vi "XY with TipTilt Z.vi"() -> ()   [LabVIEW 2012]
uses:
  Madlib.dll
panel:
  in  "X axis":dbl caption="X axis (um)" format="%.3f"
  in  "Y axis (um)":dbl format="%.3f"
  in  "?":bool
  out "Read Theta A 2":dbl format="%.3f"
  out "Read Theta B 2":dbl format="%.3f"
  out "Min. Z-Axis (um)":dbl format="%.4f"
  out "Max. Z-Axis (um)":dbl format="%.4f"
  out "Theta Y (mrad)":dbl format="%.4f"
  out "Theta X (mrad)":dbl format="%.4f"
  in  "Theta Y (mrad)":dbl format="%.4f"
  out "Center (um)":dbl format="%.4f"
  in  "Z axis (um)":dbl=50.0 format="%.4f"
  in  "Theta X (mrad)":dbl format="%.4f"
  out "Min. Theta Y (mrad)":dbl format="%.4f"
  out "Max. Theta Y (mrad)":dbl format="%.4f"
  out "Min. Theta X (mrad)":dbl format="%.4f"
  out "Max. Theta X (mrad)":dbl format="%.4f"
  out "Read Theta C":dbl caption="C (um)" format="%.3f"
  out "Read Theta B":dbl caption="B (um)" format="%.3f"
  out "Read Theta A":dbl caption="A (um)" format="%.3f"
  in  "?":bool
  # "Note: You will need to obtain a handle to each controller\nusing GetHandleByType.vi to distinguish between the \ncontrollers. The initial type values passed to this VI  may\n have to be changed to work with your controllers."
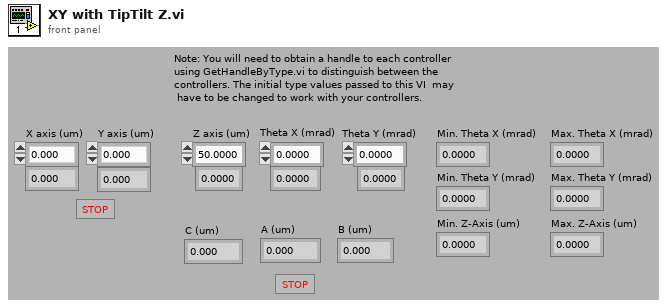
[diagram p1: front panel]
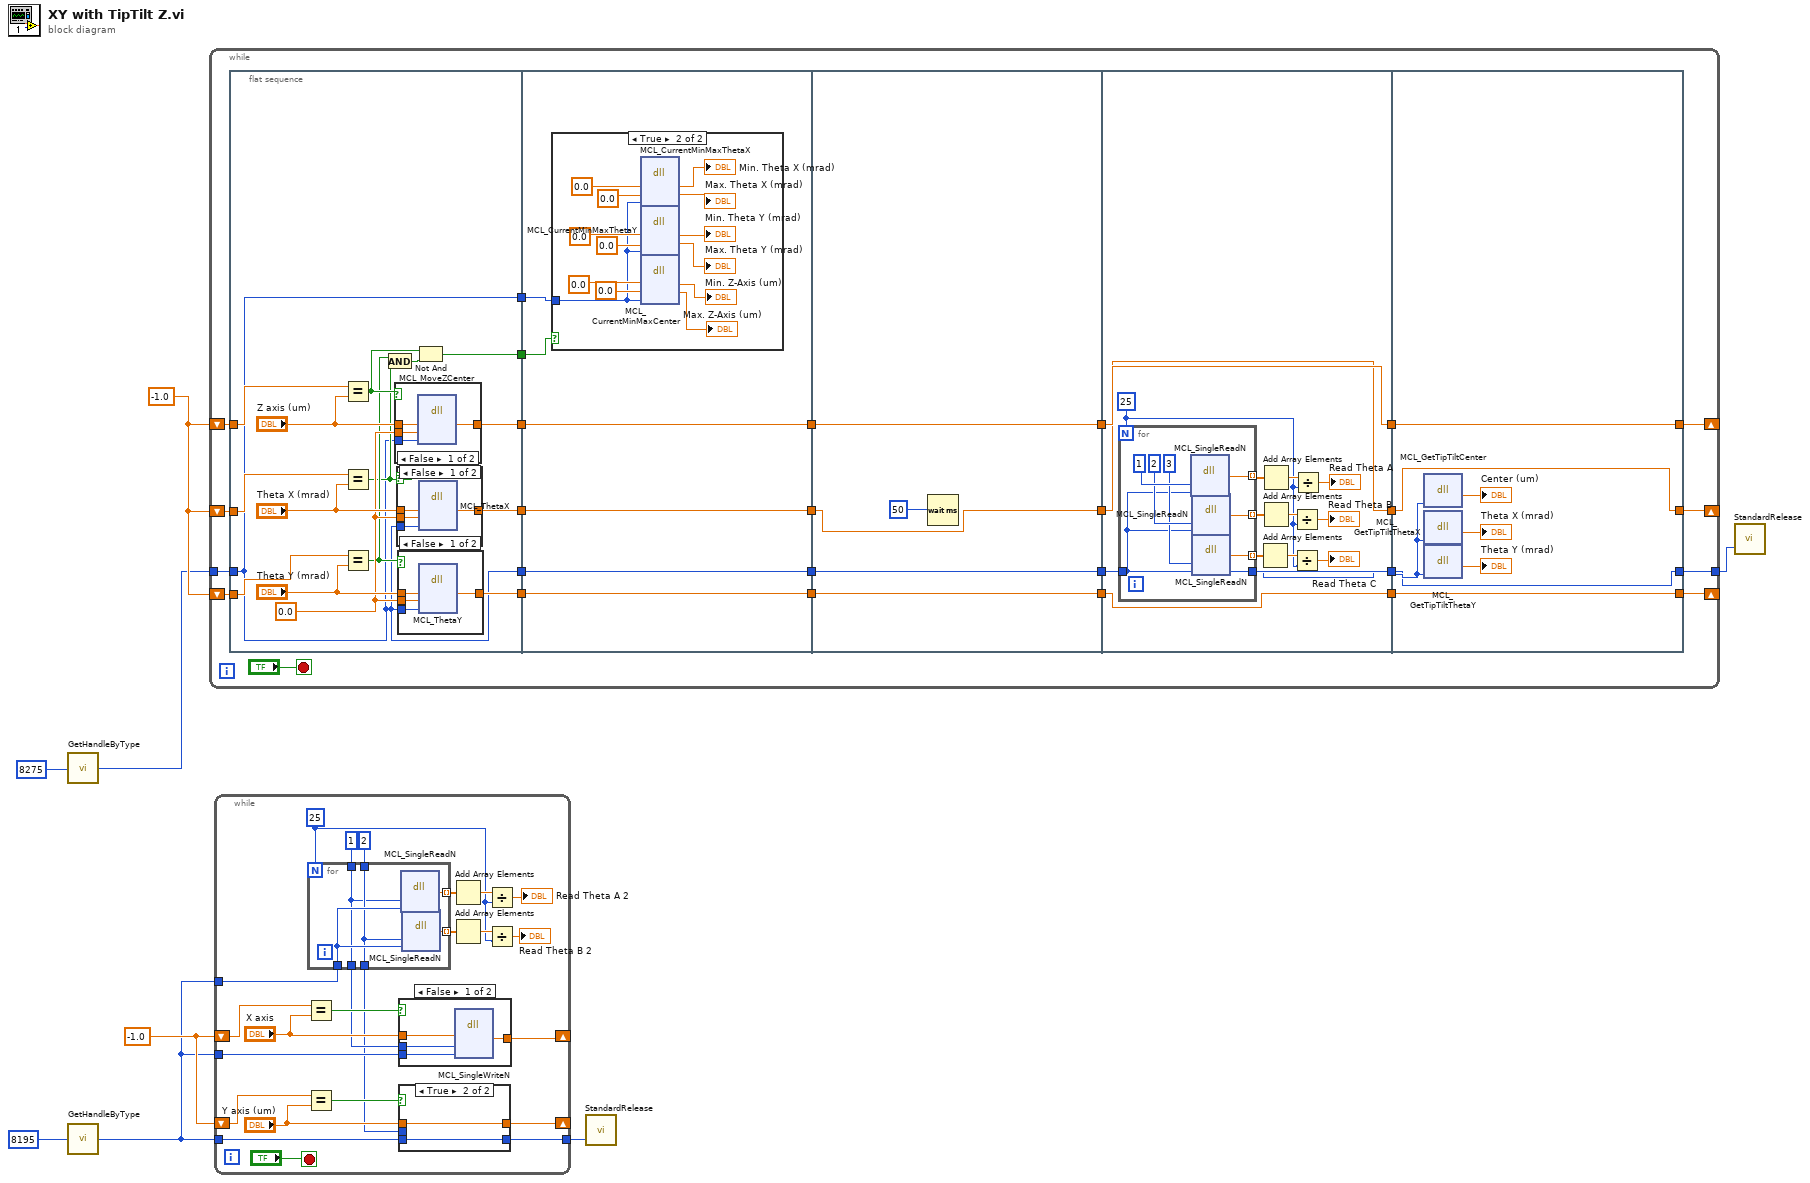
[diagram p0: block diagram]
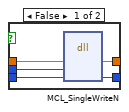
[diagram p2: hidden frame]
diagram:
  w5 = -1.0
  w7 = -1.0
  n1 = call "GetHandleByType.vi"("Type"=8275) -> ("Handle"=w6:i32)
  n2 = call "GetHandleByType.vi"("Type"=8195) -> ("Handle"=w2:i32)
  n3 = while {
    tunnel: w6 -> [w36]
    tunnel: [w35] -> w8
    shift-right: [w31] -> _
    shift-left: w7 -> [w30]
    shift-right: [w29] -> _
    shift-left: w7 -> [w28]
    shift-right: [w32] -> _
    shift-left: w7 -> [w33]
    stop <- "?" stop-if-true
    n4 = flat-sequence {
      tunnel: w36 -> [w38]
      tunnel: [w38] -> w27
      tunnel: w33 -> [w52]
      tunnel: [w50] -> w26
      tunnel: [w49] -> w25
      tunnel: w30 -> [w48]
      tunnel: [w46] -> w24
      tunnel: w28 -> [w45]
      tunnel: [w37] -> w10
      tunnel: [w38] -> w9
      tunnel: w27 -> [w73]
      tunnel: [w73] -> w23
      tunnel: w26 -> [w72]
      tunnel: [w72] -> w22
      tunnel: w25 -> [w71]
      tunnel: [w71] -> w21
      tunnel: w24 -> [w70]
      tunnel: [w70] -> w20
      tunnel: w10 -> [w69]
      tunnel: w9 -> [w68]
      tunnel: w23 -> [w90]
      tunnel: [w90] -> w19
      tunnel: w22 -> [w89]
      tunnel: [w89] -> w18
      tunnel: w21 -> [w88]
      tunnel: [w88] -> w17
      tunnel: w20 -> [w87]
      tunnel: [w87] -> w16
      tunnel: w19 -> [w106]
      tunnel: [w106] -> w15
      tunnel: [w105] -> w14
      tunnel: w18 -> [w94]
      tunnel: [w94] -> w13
      tunnel: w17 -> [w93]
      tunnel: [w93] -> w12
      tunnel: w16 -> [w92]
      tunnel: [w92] -> w11
      tunnel: w15 -> [w119]
      tunnel: [w118] -> w35
      tunnel: w14 -> [w118]
      tunnel: [w117] -> w32
      tunnel: w13 -> [w117]
      tunnel: [w116] -> w31
      tunnel: w12 -> [w116]
      tunnel: [w115] -> w29
      tunnel: w11 -> [w115]
      frame #0 {
        w43 = 0.0
        n5 = Equal?(x=w52, y="Z axis (um)") -> (x = y?=w42:bool)
        n6 = Equal?(x=w48, y="Theta X (mrad)") -> (x = y?=w40:bool)
        n7 = Equal?(x=w45, y="Theta Y (mrad)") -> (x = y?=w41:bool)
        n8 = And(x=w41, y=w40) -> (x .and. y?=w39:bool)
        n9 = case shown="False" w42 {
          tunnel: "Z axis (um)" -> [w66 w67]
          tunnel: [w65 w67] -> w50
          tunnel: w43 -> [w64 _]
          tunnel: w38 -> [w63 _]
          frame False {
            n10 = dll-call lib="C:/Users/Labview/Desktop/SRR/Madlib_x64/Labview Examples/MADLib.dll" fn="MCL_MoveZCenter"("center"=w66, "actual"=w64, "handle"=w63) -> ("center"=w65:dbl)  [unwired: 6 in, 2 out]
          }
          frame True {
          }
        }
        n11 = case shown="False" w40 {
          tunnel: [w61 w62] -> w49
          tunnel: "Theta X (mrad)" -> [w60 w62]
          tunnel: w43 -> [w59 _]
          tunnel: w38 -> [w58 _]
          frame False {
            n12 = dll-call lib="C:/Users/Labview/Desktop/SRR/Madlib_x64/Labview Examples/MADLib.dll" fn="MCL_ThetaX"("milliradians"=w60, "actual"=w59, "handle"=w58) -> ("milliradians"=w61:dbl)  [unwired: 6 in, 2 out]
          }
          frame True {
          }
        }
        n13 = case shown="False" w41 {
          tunnel: [w56 w57] -> w46
          tunnel: "Theta Y (mrad)" -> [w55 w57]
          tunnel: w43 -> [w54 _]
          tunnel: w38 -> [w53 _]
          frame False {
            n14 = dll-call lib="C:/Users/Labview/Desktop/SRR/Madlib_x64/Labview Examples/MADLib.dll" fn="MCL_ThetaY"("milliradians"=w55, "actual"=w54, "handle"=w53) -> ("milliradians"=w56:dbl)  [unwired: 6 in, 2 out]
          }
          frame True {
          }
        }
        n15 = Not And(1:w39, 2:w42) -> (0:w37:bool)
      }
      frame #1 {
        n16 = case shown="True" w69 {
          tunnel: w68 -> [_ w74]
          frame False {
          }
          frame True {
            n17 = dll-call lib="C:/Users/Labview/Desktop/SRR/Madlib_x64/Labview Examples/MADLib.dll" fn="MCL_CurrentMinMaxThetaX"("min"=0.0, "max"=0.0, "handle"=w74) -> ("min"=→"Min. Theta X (mrad)":dbl, "max"=→"Max. Theta X (mrad)":dbl)  [unwired: 5 in, 2 out]
            n18 = dll-call lib="C:/Users/Labview/Desktop/SRR/Madlib_x64/Labview Examples/MADLib.dll" fn="MCL_CurrentMinMaxThetaY"("min"=0.0, "max"=0.0, "handle"=w74) -> ("min"=→"Min. Theta Y (mrad)":dbl, "max"=→"Max. Theta Y (mrad)":dbl)  [unwired: 5 in, 2 out]
            n19 = dll-call lib="C:/Users/Labview/Desktop/SRR/Madlib_x64/Labview Examples/MADLib.dll" fn="MCL_CurrentMinMaxCenter"("min"=0.0, "max"=0.0, "handle"=w74) -> ("min"=→"Min. Z-Axis (um)":dbl, "max"=→"Max. Z-Axis (um)":dbl)  [unwired: 5 in, 2 out]
          }
        }
      }
      frame #2 {
        n20 = Wait (ms)(milliseconds to wait=50) -> ()  [unwired: 1 out]
      }
      frame #3 {
        w98 = 25
        n21 = for {
          N: w98 -> [_]
          tunnel: [w111] -> w102 mode=indexing
          tunnel: [w110] -> w104 mode=indexing
          tunnel: [w109] -> w103 mode=indexing
          tunnel: w106 -> [w108]
          tunnel: [w107] -> w105
          n22 = dll-call lib="C:/Users/Labview/Desktop/SRR/Madlib_x64/Labview Examples/MADLib.dll" fn="MCL_SingleReadN"("axis"=1, "handle"=w108) -> (w111:dbl)  [unwired: 5 in, 2 out]
          n23 = dll-call lib="C:/Users/Labview/Desktop/SRR/Madlib_x64/Labview Examples/MADLib.dll" fn="MCL_SingleReadN"("axis"=2, "handle"=w108) -> (w110:dbl)  [unwired: 5 in, 2 out]
          n24 = dll-call lib="C:/Users/Labview/Desktop/SRR/Madlib_x64/Labview Examples/MADLib.dll" fn="MCL_SingleReadN"("axis"=3, "handle"=w108) -> (w109:dbl, "handle"=w107:i32)  [unwired: 4 in, 2 out]
        }
        n25 = Add Array Elements(numeric array=w103) -> (sum=w99:dbl)
        n26 = Add Array Elements(numeric array=w102) -> (sum=w101:dbl)
        n27 = Add Array Elements(numeric array=w104) -> (sum=w100:dbl)
        n28 = Divide(x=w100, y=w98) -> (x/y=→"Read Theta B":dbl)
        n29 = Divide(x=w99, y=w98) -> (x/y=→"Read Theta C":dbl)
        n30 = Divide(x=w101, y=w98) -> (x/y=→"Read Theta A":dbl)
      }
      frame #4 {
        n31 = dll-call lib="C:/Users/Labview/Desktop/SRR/Madlib_x64/Labview Examples/MADLib.dll" fn="MCL_GetTipTiltCenter"("handle"=w119) -> (→"Center (um)":dbl)  [unwired: 4 in, 2 out]
        n32 = dll-call lib="C:/Users/Labview/Desktop/SRR/Madlib_x64/Labview Examples/MADLib.dll" fn="MCL_GetTipTiltThetaX"("handle"=w119) -> (→"Theta X (mrad)":dbl)  [unwired: 4 in, 2 out]
        n33 = dll-call lib="C:/Users/Labview/Desktop/SRR/Madlib_x64/Labview Examples/MADLib.dll" fn="MCL_GetTipTiltThetaY"("handle"=w119) -> (→"Theta Y (mrad)":dbl)  [unwired: 4 in, 2 out]
      }
    }
  }
  n34 = while {
    shift-right: [w144] -> _
    shift-left: w5 -> [w146]
    shift-right: [w143] -> _
    shift-left: w5 -> [w145]
    tunnel: w2 -> [w138]
    tunnel: w2 -> [w137]
    tunnel: w2 -> [w133]
    tunnel: [w123] -> w1
    stop <- "?" stop-if-true
    w124 = 25
    n35 = Equal?(x=w146, y="X axis") -> (x = y?=w139:bool)
    n36 = Equal?(x=w145, y="Y axis (um)") -> (x = y?=w142:bool)
    n37 = for {
      N: w124 -> [_]
      tunnel: [w147] -> w135
      tunnel: [w148] -> w134
      tunnel: w133 -> [w151]
      tunnel: [w150] -> w129 mode=indexing
      tunnel: [w149] -> w130 mode=indexing
      tunnel: 2 -> [w148]
      tunnel: 1 -> [w147]
      n38 = dll-call lib="C:/Users/Labview/Desktop/SRR/Madlib_x64/Labview Examples/MADLib.dll" fn="MCL_SingleReadN"("axis"=w147, "handle"=w151) -> (w150:dbl)  [unwired: 5 in, 2 out]
      n39 = dll-call lib="C:/Users/Labview/Desktop/SRR/Madlib_x64/Labview Examples/MADLib.dll" fn="MCL_SingleReadN"("axis"=w148, "handle"=w151) -> (w149:dbl)  [unwired: 5 in, 2 out]
    }
    n40 = case shown="False" w139 {
      tunnel: [w162 w163] -> w144
      tunnel: "X axis" -> [w161 w163]
      tunnel: w138 -> [w160 _]
      tunnel: w135 -> [w159 _]
      frame False {
        n41 = dll-call lib="C:/Users/Labview/Desktop/SRR/Madlib_x64/Labview Examples/MADLib.dll" fn="MCL_SingleWriteN"("position"=w161, "axis"=w159, "handle"=w160) -> ("position"=w162:dbl)  [unwired: 6 in, 2 out]
      }
      frame True {
      }
    }
    n42 = case shown="True" w142 {
      tunnel: [w156 w158] -> w143
      tunnel: "Y axis (um)" -> [w155 w158]
      tunnel: w137 -> [w154 w157]
      tunnel: w134 -> [w153 _]
      tunnel: [w152 w157] -> w123
      frame False {
        n43 = dll-call lib="C:/Users/Labview/Desktop/SRR/Madlib_x64/Labview Examples/MADLib.dll" fn="MCL_SingleWriteN"("position"=w155, "axis"=w153, "handle"=w154) -> ("position"=w156:dbl, "handle"=w152:i32)  [unwired: 5 in, 2 out]
      }
      frame True {
      }
    }
    n44 = Add Array Elements(numeric array=w129) -> (sum=w128:dbl)
    n45 = Add Array Elements(numeric array=w130) -> (sum=w127:dbl)
    n46 = Divide(x=w128, y=w124) -> (x/y=→"Read Theta A 2":dbl)
    n47 = Divide(x=w127, y=w124) -> (x/y=→"Read Theta B 2":dbl)
  }
  n48 = call "StandardRelease.vi"("Outgoing Handle"=w1) -> ()  [unwired: 2 in]
  n49 = call "StandardRelease.vi"("Outgoing Handle"=w8) -> ()  [unwired: 2 in]
